vi "SaveImageFile.vi"(8 "error in":errorcluster, 9 "ImagData":u8[](array[numeric])=array[1228800 elements] format="%x", 10 "FileName":string="TestImage") -> (0 "error out":errorcluster, 2 "appended path":path, 3 "success?":bool=TRUE)   [LabVIEW 2014]
panel:
  out "Right":i32=1280
  out "Bottom":i32=960
  out "Cal size":u64=1229878
  in  "Left":i16
  in  "Top":i16
  in  "Right":u16=1280
  in  "Bottom":u16=960
  out "picture":picture
  out "out cluster":T1={0, 8, "ImagData"=array[1229878 elements], [], [0, 65793, 131586, 197379, 263172, 328965, 394758, 460551, 526344, 592137, 657930, 723723, 789516, 855309, 921102, 986895, 1052688, 1118481, 1184274, 1250067, 1315860, 1381653, 1447446, 1513239, 1579032, 1644825, 1710618, 1776411, 1842204, 1907997, 1973790, 2039583, 2105376, 2171169, 2236962, 2302755, 2368548, 2434341, 2500134, 2565927, 2631720, 2697513, 2763306, 2829099, 2894892, 2960685, 3026478, 3092271, 3158064, 3223857, 3289650, 3355443, 3421236, 3487029, 3552822, 3618615, 3684408, 3750201, 3815994, 3881787, 3947580, 4013373, 4079166, 4144959, 4210752, 4276545, 4342338, 4408131, 4473924, 4539717, 4605510, 4671303, 4737096, 4802889, 4868682, 4934475, 5000268, 5066061, 5131854, 5197647, 5263440, 5329233, 5395026, 5460819, 5526612, 5592405, 5658198, 5723991, 5789784, 5855577, 5921370, 5987163, 6052956, 6118749, 6184542, 6250335, 6316128, 6381921, 6447714, 6513507, 6579300, 6645093, 6710886, 6776679, 6842472, 6908265, 6974058, 7039851, 7105644, 7171437, 7237230, 7303023, 7368816, 7434609, 7500402, 7566195, 7631988, 7697781, 7763574, 7829367, 7895160, 7960953, 8026746, 8092539, 8158332, 8224125, 8289918, 8355711, 8421504, 8487297, 8553090, 8618883, 8684676, 8750469, 8816262, 8882055, 8947848, 9013641, 9079434, 9145227, 9211020, 9276813, 9342606, 9408399, 9474192, 9539985, 9605778, 9671571, 9737364, 9803157, 9868950, 9934743, 10000536, 10066329, 10132122, 10197915, 10263708, 10329501, 10395294, 10461087, 10526880, 10592673, 10658466, 10724259, 10790052, 10855845, 10921638, 10987431, 11053224, 11119017, 11184810, 11250603, 11316396, 11382189, 11447982, 11513775, 11579568, 11645361, 11711154, 11776947, 11842740, 11908533, 11974326, 12040119, 12105912, 12171705, 12237498, 12303291, 12369084, 12434877, 12500670, 12566463, 12632256, 12698049, 12763842, 12829635, 12895428, 12961221, 13027014, 13092807, 13158600, 13224393, 13290186, 13355979, 13421772, 13487565, 13553358, 13619151, 13684944, 13750737, 13816530, 13882323, 13948116, 14013909, 14079702, 14145495, 14211288, 14277081, 14342874, 14408667, 14474460, 14540253, 14606046, 14671839, 14737632, 14803425, 14869218, 14935011, 15000804, 15066597, 15132390, 15198183, 15263976, 15329769, 15395562, 15461355, 15527148, 15592941, 15658734, 15724527, 15790320, 15856113, 15921906, 15987699, 16053492, 16119285, 16185078, 16250871, 16316664, 16382457, 16448250, 16514043, 16579836, 16645629, 16711422, 16777215], {0, 0, 1280, 960}}
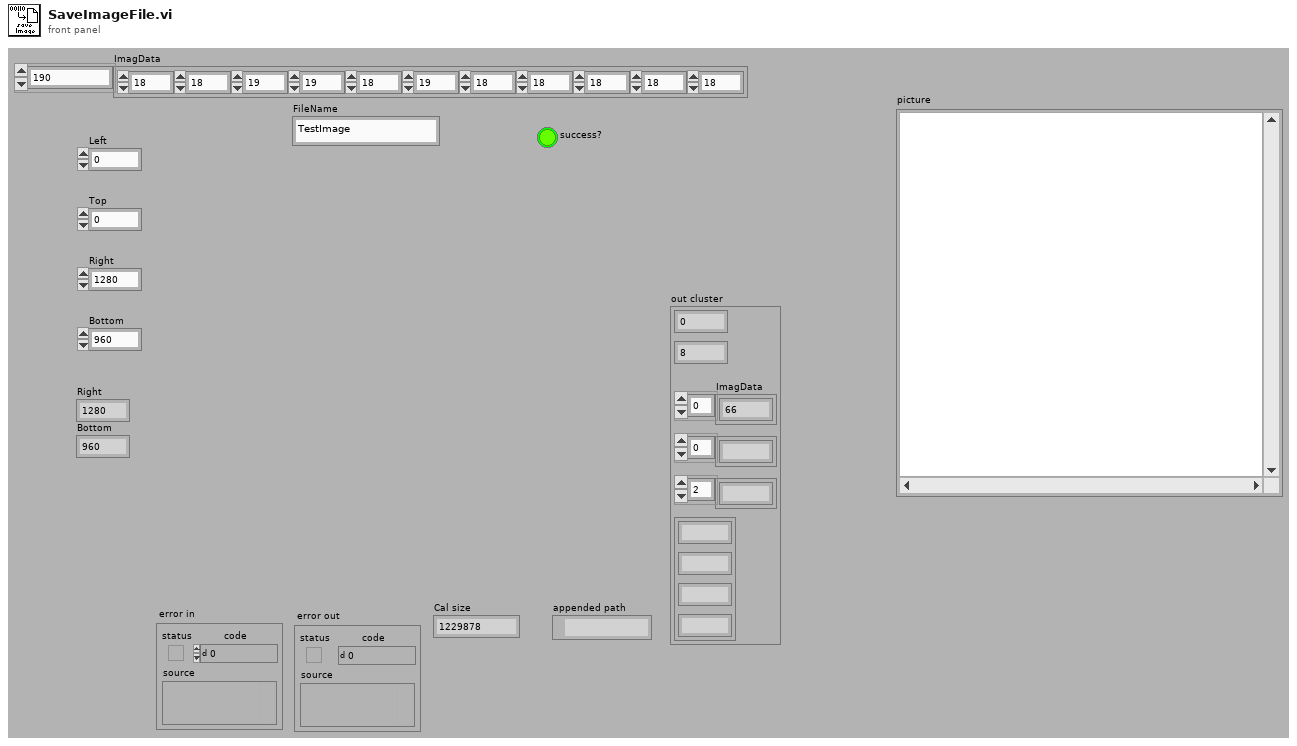
[diagram p1: front panel]
types:
  T1 = cluster{u16, u8, "ImagData":u8[], u8[], i32[], cluster{i16, i16, u16, u16}}
  T2 = cluster{u16, u8, u8[], u8[], i32[], cluster{i32, i32, u16, u16}}
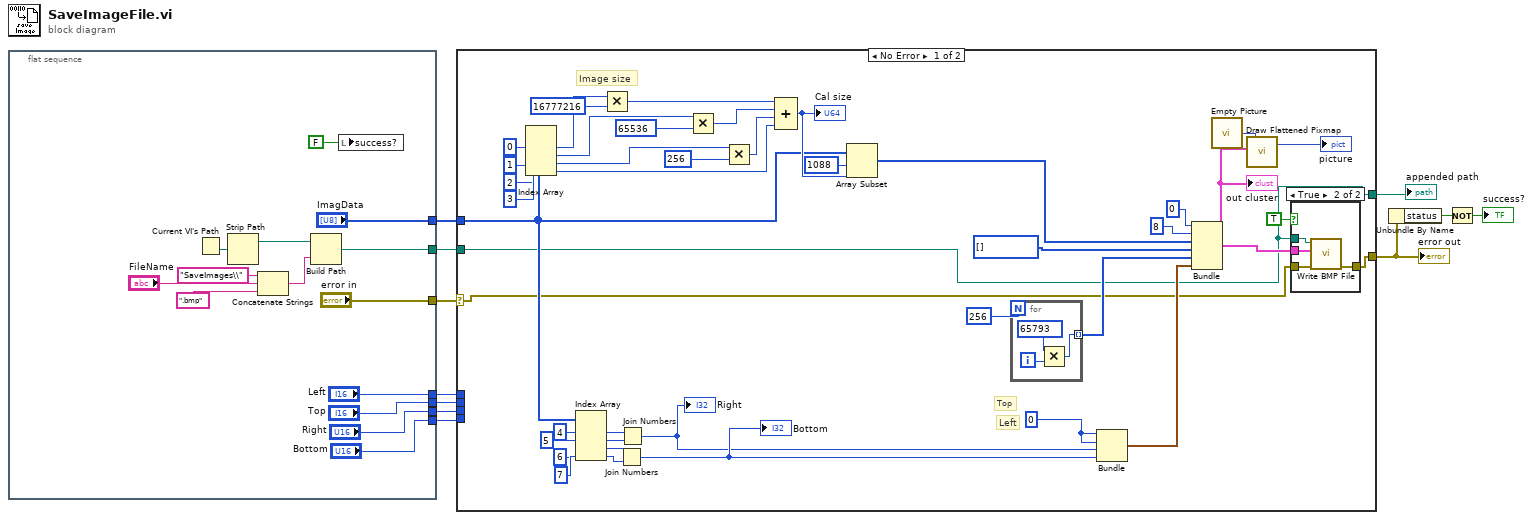
[diagram p0: block diagram]
diagram:
  n1 = flat-sequence {
    tunnel: ["Left"] -> w11
    tunnel: ["Top"] -> w10
    tunnel: ["Right"] -> w9
    tunnel: ["Bottom"] -> w8
    tunnel: ["ImagData"] -> w7
    tunnel: ["error in"] -> w6
    tunnel: [w14] -> w3
    frame #0 {
      n2 = Current VI's Path() -> (path=w19:path)
      n3 = Strip Path(path=w19) -> (stripped path=w18:path)  [unwired: 1 out]
      n4 = Concatenate Strings("SaveImages\\" ("string"), "FileName", ".bmp" ("string")) -> (w17:string)
      n5 = Build Path(base path=w18, name or relative path=w17) -> (appended path=w14:path)
      n6 = local write "success?"(FALSE ("success?")) -> ()
    }
  }
  n7 = case shown="No Error" w6 {
    selector: w6 -> [w31 w76]
    tunnel: w11 -> [_ _]
    tunnel: w10 -> [_ _]
    tunnel: w9 -> [_ _]
    tunnel: w8 -> [_ _]
    tunnel: w7 -> [w34 _]
    tunnel: [w60 w76] -> w2
    tunnel: w3 -> [w27 _]
    tunnel: [w27 _] -> w1
    frame No Error {
      w30 = 0
      # "Left"
      # "Top"
      # "Image size"
      n8 = Index Array(array=w34, index #1=0 ("index"), index #2=1 ("index"), index #3=2 ("index"), index #4=3 ("index")) -> (element #1=w49:u8, element #2=w52:u8, element #3=w54:u8, element #4=w58:u8)
      n9 = Index Array(array=w34, index #1=4 ("index"), index #2=5 ("index"), index #3=6 ("index"), index #4=7 ("index")) -> (element #1=w39:u8, element #2=w40:u8, element #3=w41:u8, element #4=w42:u8)
      n10 = Multiply(x=w49, y=u64 16777216) -> (x*y=w55:u64)
      n11 = Join Numbers(hi=w41, lo=w42) -> ((hi.lo)=w29:u16)
      "Bottom" <- w29
      n12 = Join Numbers(hi=w39, lo=w40) -> ((hi.lo)=w28:u16)
      "Right" <- w28
      n13 = Multiply(x=w52, y=u64 65536) -> (x*y=w56:u64)
      n14 = Multiply(x=w54, y=u64 256) -> (x*y=w57:u64)
      n15 = Compound Arithmetic op=ADD(w55, w56, w57, w58) -> (w43:u64)
      "Cal size" <- w43
      n16 = Array Subset(array=w34, index=1088, length=w43) -> (w32:u8[])
      n17 = for {
        N: 256 -> [_]
        tunnel: [w73] -> w59 mode=indexing
        i -> [w74]
        n18 = Multiply(x=65793, y=w74) -> (x*y=w73:i32)
      }
      n19 = Bundle(w30, w30, w28, w29) -> (w67:cluster{i32, i32, u16, u16})  [unwired: 1 in]
      n20 = Bundle(u16 0, u8 8, w32, u8[] [], w59, w67) -> (w63:T2)  [unwired: 1 in]
      "out cluster" <- w63
      n21 = call "Empty Picture"() -> ("empty picture"=w61:picture)
      n22 = call <vilib>:"Draw Flattened Pixmap.vi"("image data"=w63, "picture"=w61) -> ("new picture"=→"picture":picture)  [unwired: 7 in]
      n23 = case shown="True" TRUE {
        tunnel: w63 -> [_ w72]
        tunnel: [w68 w71] -> w60
        tunnel: w31 -> [w68 w70]
        tunnel: w27 -> [_ w69]
        frame False {
        }
        frame True {
          n24 = call <vilib>:"Write BMP File.vi"("error in (no error)"=w70, "image data"=w72, "path to BMP file"=w69) -> ("error out"=w71:errorcluster)  [unwired: 7 in, 1 out]
        }
      }
    }
    frame Error {
    }
  }
  "error out" <- w2
  "appended path" <- w1
  n25 = Unbundle By Name(w2) -> ("status"=w5:bool)
  n26 = Not(x=w5) -> (.not. x?=→"success?":bool)
